vi "Comm@Read__Parameter.vi"(1 "ParamterIn":string) -> (0 "ParamterOut":string)   [LabVIEW 2020]
panel:
  in  "Message":string(combo)
  in  "Number":string(combo)
  in  "Variable":string(combo)
  in  "CommName":string(combo)
  in  "Confirm":bool
  # "Comm@Read $Comm,$Variable,$Number(,$[[label]]Message)"
  # "COM               $Variable,$Number,$[[label]]Message)\nTCP                $Variable,$Number,$[[label]]Message)\nListen              $Variable,$Number,$[[label]]Message)\nModbus           $Variable,$Address(:$Number)(,$[[label]]Message)\nModbus(TCP)   $Variable,$Address(:$Number)(,$[[label]]Message)"
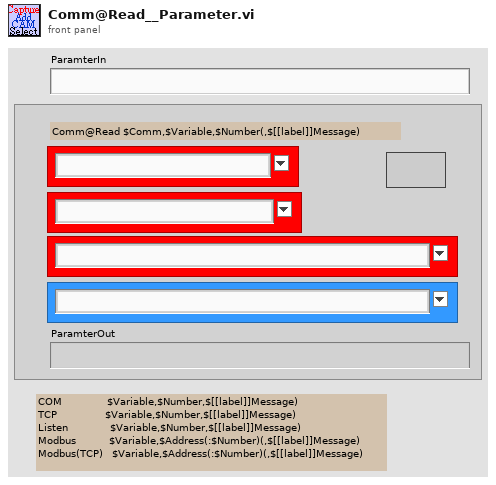
[diagram p1: front panel]
types:
  T1 = enum16{"Get", "Init", "Set", "Delete", "GetElement", "Inc", "Dec", "ReName"}
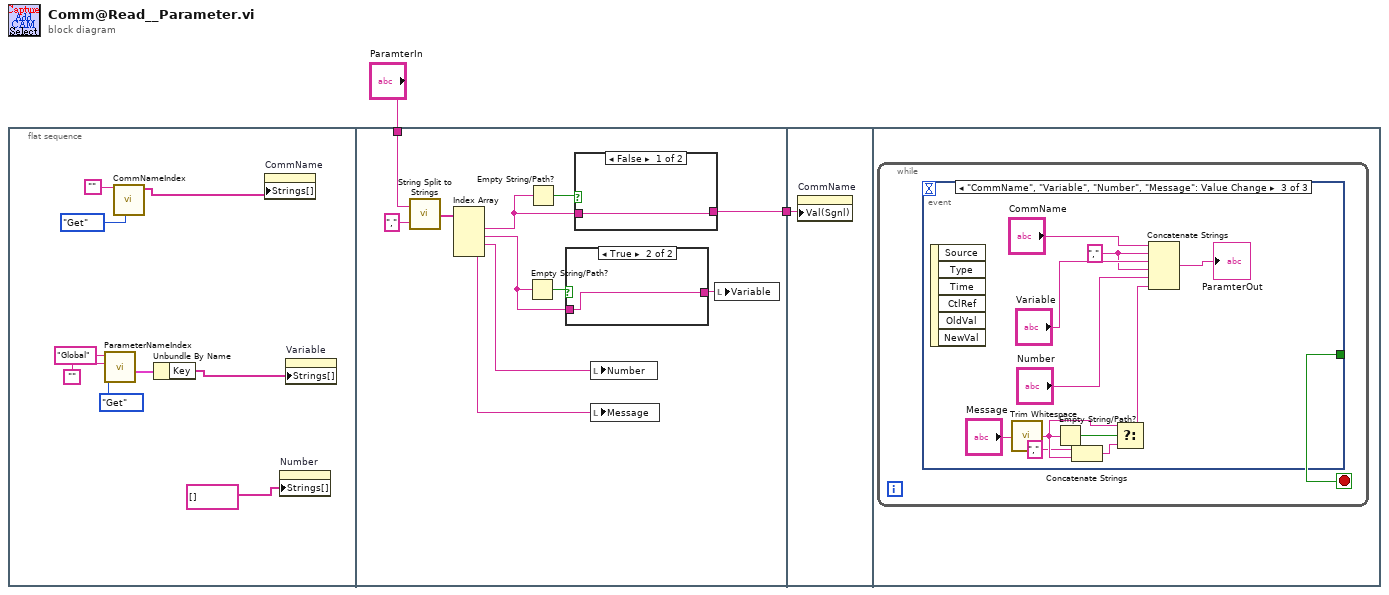
[diagram p0: block diagram]
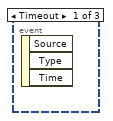
[diagram p4: hidden frame]
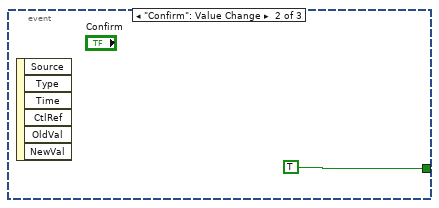
[diagram p5: hidden frame]
diagram:
  n1 = flat-sequence {
    tunnel: "ParamterIn" -> [w18]
    tunnel: [w20] -> w1
    tunnel: w1 -> [w27]
    frame #0 {
      n2 = call "ParameterNameIndex.vi"("OP"=T1."Get", "Key"="", "VariableSection"="Global") -> ("GlobalKeyValue"=w7:cluster{"Key":string[], "Value":string[]})  [unwired: 2 in, 6 out]
      n3 = call "CommNameIndex.vi"("OP"=enum16{"Init", "Get", "Set"}."Get", "Comm"="") -> ("CommNameS"=w9:string[])  [unwired: 7 in, 2 out]
      n4 = Unbundle By Name(w7) -> ("Key"=w6:string[])
      n5 = property on="CommName" class="CmbBox"("Strings[]"=w9) -> ()  [unwired: 2 in, 2 out]
      n6 = property on="Number" class="CmbBox"("Strings[]"=string[] [] ("Strings []")) -> ()  [unwired: 2 in, 2 out]
      n7 = property on="Variable" class="CmbBox"("Strings[]"=w6) -> ()  [unwired: 2 in, 2 out]
    }
    frame #1 {
      n8 = call "String Split to Strings.vi"("search string/char (-)"=",", "String"=w18) -> ("Array"=w16:string[])
      n9 = Index Array(array=w16) -> (element #1=w15:string, element #2=w14:string, element #3=w13:string, element #4=w12:string)  [unwired: 4 in]
      n10 = Empty String/Path?(string/path=w14) -> (empty?=w21:bool)
      n11 = Empty String/Path?(string/path=w15) -> (empty?=w22:bool)
      n12 = case shown="True" w21 {
        tunnel: w14 -> [w23 w24]
        tunnel: [w23 w24] -> w19
        frame False {
        }
        frame True {
        }
      }
      n13 = case shown="False" w22 {
        tunnel: [w25 w26] -> w20
        tunnel: w15 -> [w25 w26]
        frame False {
        }
        frame True {
        }
      }
      n14 = local write "Number"(w13) -> ()
      n15 = local write "Message"(w12) -> ()
      n16 = local write "Variable"(w19) -> ()
    }
    frame #2 {
      n17 = property on="CommName" class="CmbBox"("Val(Sgnl)"=w27) -> ()  [unwired: 2 in, 2 out]
    }
    frame #3 {
      n18 = while {
        stop <- w28 stop-if-true
        n19 = event shown="[2] \"CommName\", \"Variable\", \"Number\", \"Message\": Value Change" {
          selector: _ -> [_ _ _]
          dyn-events: _ -> [_ _ _]
          timeout: _ -> [_ _ _]
          tunnel: [_ TRUE _] -> w28
          event Timeout {
            n20 = event-data() -> ()  [unwired: 1 in, 3 out]
          }
          event "Confirm": Value Change {
            n21 = event-data() -> ()  [unwired: 1 in, 6 out]
          }
          event "CommName", "Variable", "Number", "Message": Value Change {
            w36 = "," ("string")
            n22 = event-data() -> ()  [unwired: 1 in, 6 out]
            n23 = call <vilib>:"Trim Whitespace.vi"("string"="Message") -> ("trimmed string"=w33:string)  [unwired: 1 in]
            n24 = Empty String/Path?(string/path=w33) -> (empty?=w34:bool)
            n25 = Concatenate Strings("," ("string"), w33) -> (w30:string)
            n26 = Select(t=w33, s=w34, f=w30) -> (s? t:f=w31:string)
            n27 = Concatenate Strings("CommName", w36, "Variable", w36, "Number", w31) -> (→"ParamterOut":string)
          }
        }
      }
    }
  }
